vi "NATS READ.vi"(6 "timeout ms (conn default)":i32=-2, 7 "bytes to read (1024)":i32=1024, 8 "error in":errorcluster, 9 "reread on PING? (T)":bool=TRUE, 10 "suppress timeout error? (T)":bool=TRUE, 11 "nats connection in":T3={"connection ID"=refnum, "server INFO"="", "timeout ms"=5000, "verbose?"=FALSE, "server headers?"=FALSE, "client headers?"=FALSE}) -> (0 "error out":errorcluster, 1 "timeout?":bool, 2 "nats message":T1, 3 "nats connection out":T3={"connection ID"=refnum, "server INFO"="", "timeout ms"=5000, "verbose?"=FALSE, "server headers?"=FALSE, "client headers?"=FALSE})   [LabVIEW 2013, in "NATS Core.lvlib"]
doc: "Reads a message from the NATS server."
uses:
  NATS Core.lvlib
  Controls/nats connection.ctl
  Controls/nats message.ctl
  Controls/msg type.ctl
  <vilib>/dlg_ctls.llb/Space Constant.vi
  <vilib>/Utility/error.llb/Trim Whitespace.vi
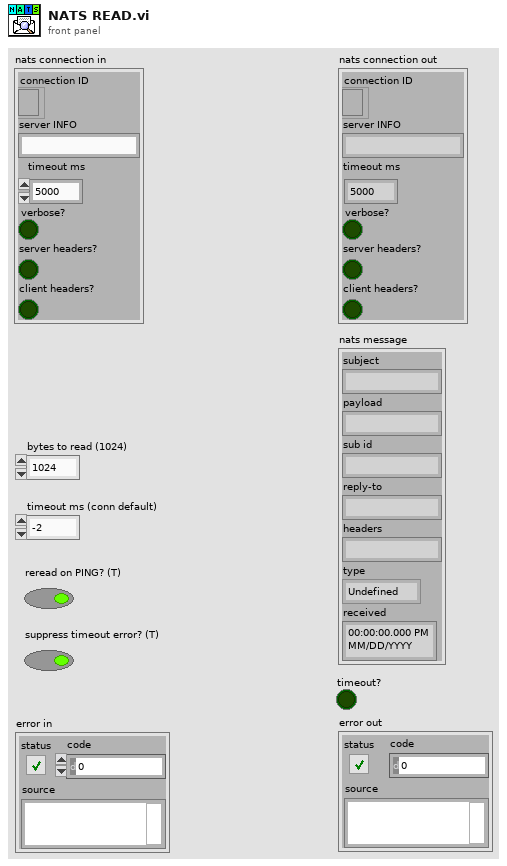
[diagram p1: front panel]
types:
  T1 = typedef "NATS Core.lvlib/nats message.ctl" = cluster{"subject":string, "payload":string, "sub id":string, "reply-to":string, "headers":string, "type":T2, "received":timestamp}
  T2 = typedef "NATS Core.lvlib/msg type.ctl" = enum16{"Undefined", "MSG", "HMSG", "+OK", "PING", "PONG", "-ERR", "INFO"}
  T3 = typedef "NATS Core.lvlib/nats connection.ctl" = cluster{"connection ID":refnum<k5>, "server INFO":string, "timeout ms":i32, "verbose?":bool, "server headers?":bool, "client headers?":bool}
  T4 = enum16{"Standard", "Buffered", "CRLF", "Immediate"}
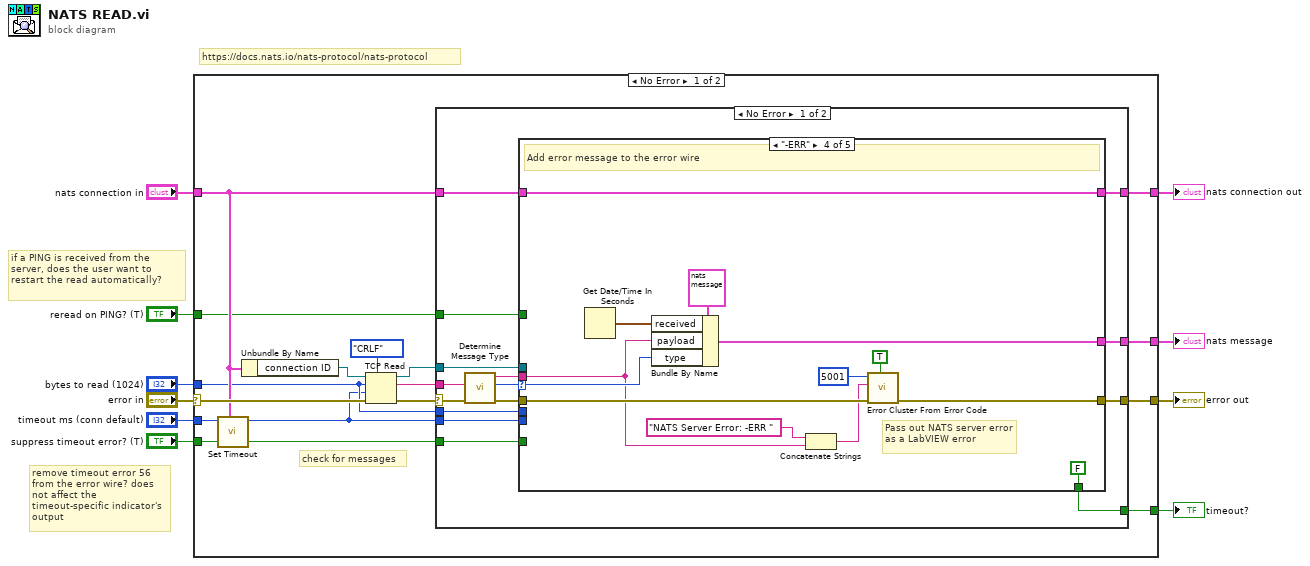
[diagram p0: block diagram]
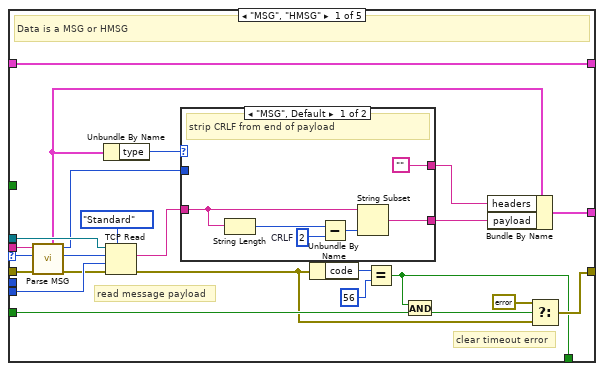
[diagram p2: hidden frame]
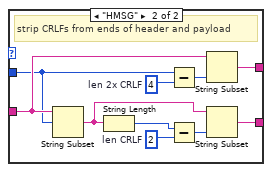
[diagram p3: hidden frame]
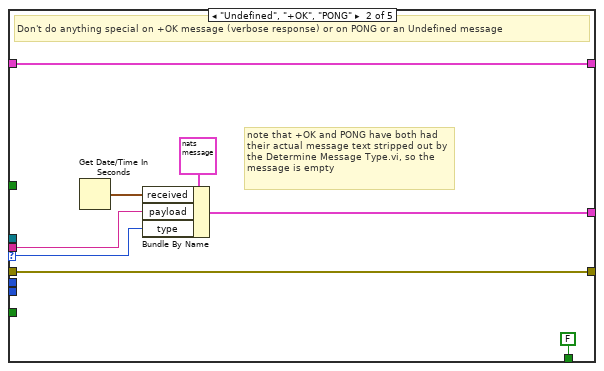
[diagram p4: hidden frame]
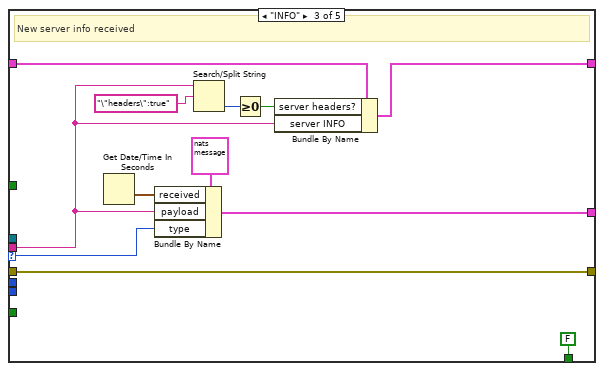
[diagram p5: hidden frame]
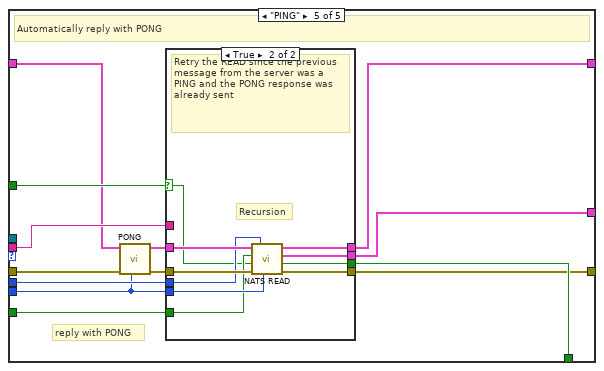
[diagram p6: hidden frame]
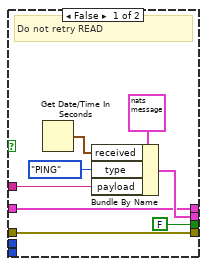
[diagram p7: hidden frame]
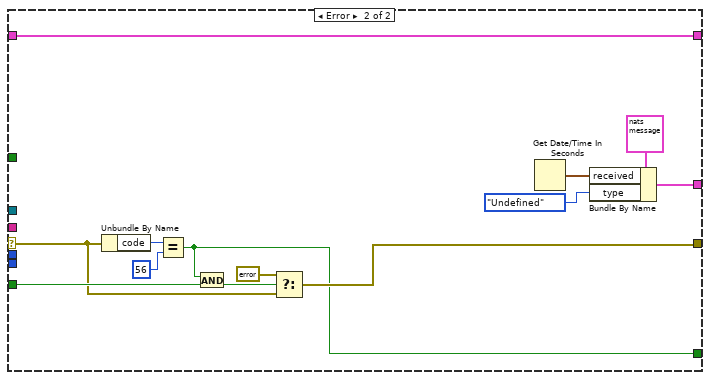
[diagram p8: hidden frame]
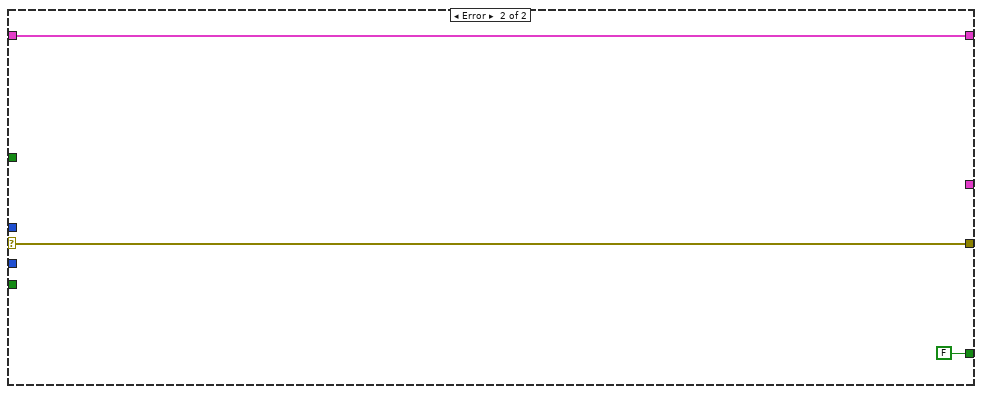
[diagram p9: hidden frame]
diagram:
  # "https://docs.nats.io/nats-protocol/nats-protocol"
  # "remove timeout error 56 from the error wire? does not affect the timeout-specific indicator's output"
  # "if a PING is received from the server, does the user want to restart the read automatically?"
  n1 = case shown="No Error" "error in" {
    selector: "error in" -> [w26 w161]
    tunnel: "nats connection in" -> [w17 w159]
    tunnel: [w24 w161] -> w8
    tunnel: "bytes to read (1024)" -> [w14 _]
    tunnel: "timeout ms (conn default)" -> [w18 _]
    tunnel: [w22 _] -> w5
    tunnel: [w21 FALSE ("specific error cleared?")] -> w4
    tunnel: [w19 w159] -> w3
    tunnel: "reread on PING? (T)" -> [w16 _]
    tunnel: "suppress timeout error? (T)" -> [w15 _]
    frame No Error {
      # "check for messages"
      n2 = call "Set Timeout.vi"("nats connection in"=w17, "timeout ms in"=w18) -> ("timeout ms out"=w13:i32)  [unwired: 9 in]
      n3 = Unbundle By Name(w17) -> ("connection ID"=w12:refnum<k5>)
      n4 = TCP Read(connection ID=w12, bytes to read=w14, error in (no error)=w26, 7:T4."CRLF" ("mode (standard)"), 9:w13) -> (connection ID out=w11:refnum<k5>, data out=w25:string, error out=w20:errorcluster)
      n5 = case shown="No Error" w20 {
        selector: w20 -> [w32 w148]
        tunnel: w25 -> [w33 _]
        tunnel: [w41 w147] -> w24
        tunnel: w13 -> [w40 _]
        tunnel: [w39 w154] -> w22
        tunnel: [w38 w146] -> w21
        tunnel: w17 -> [w37 w158]
        tunnel: [w36 w158] -> w19
        tunnel: w16 -> [w35 _]
        tunnel: w15 -> [w34 w149]
        tunnel: w14 -> [w28 _]
        tunnel: w11 -> [w27 _]
        frame No Error {
          n6 = call "Determine Message Type.vi"("error in"=w32, "data in"=w33) -> ("error out"=w31:errorcluster, "message type"=w30:T2, "stripped message"=w29:string)  [unwired: 7 in]
          n7 = case shown="\"-ERR\"" w30 {
            selector: w30 -> [w56 w88 w100 w113 _]
            tunnel: w31 -> [w53 w86 w98 w108 w118]
            tunnel: [w62 w86 w98 w107 w122] -> w41
            tunnel: w40 -> [w64 _ _ _ w115]
            tunnel: [w59 w87 w99 w112 w124] -> w39
            tunnel: [w43 FALSE ("timeout?") FALSE ("timeout?") FALSE ("timeout?") w123] -> w38
            tunnel: w37 -> [w60 w83 w90 w110 w119]
            tunnel: [w60 w83 w96 w110 w127] -> w36
            tunnel: w35 -> [_ _ _ _ w125]
            tunnel: w34 -> [w63 _ _ _ w121]
            tunnel: w29 -> [w61 w85 w93 w104 w120]
            tunnel: w28 -> [_ _ _ _ w126]
            tunnel: w27 -> [w54 _ _ _ _]
            frame "MSG", "HMSG" {
              # "clear timeout error"
              # "read message payload"
              # "Data is a MSG or HMSG"
              n8 = call "Parse MSG.vi"("error in"=w53, "message type"=w56, "stripped message"=w61) -> ("error out"=w52:errorcluster, "bytes to read"=w51:i32, "header length"=w48:i32, "nats message"=w49:T1)  [unwired: 5 in]
              n9 = Unbundle By Name(w49) -> ("type"=w50:T2)
              n10 = TCP Read(connection ID=w54, bytes to read=w51, error in (no error)=w52, 7:T4."Standard" ("mode (standard)"), 9:w64) -> (data out=w58:string, error out=w47:errorcluster)  [unwired: 1 out]
              n11 = case shown="\"MSG\", Default" w50 {
                tunnel: w58 -> [w69 w78]
                tunnel: w48 -> [_ w77]
                tunnel: ["" w79] -> w55
                tunnel: [w68 w74] -> w57
                frame "MSG", Default {
                  w67 = 2  # CRLF
                  # "strip CRLF from end of payload"
                  n12 = String Length(string=w69) -> (length=w66:i32)
                  n13 = Subtract(x=w66, y=w67) -> (x-y=w70:i32)
                  n14 = String Subset(string=w69, length (rest)=w70) -> (substring=w68:string)  [unwired: 1 in]
                }
                frame "HMSG" {
                  w76 = 2  # len CRLF
                  w80 = 4  # len 2x CRLF
                  # "strip CRLFs from ends of header and payload"
                  n15 = String Subset(string=w78, offset (0)=w77) -> (substring=w72:string)  [unwired: 1 in]
                  n16 = String Length(string=w72) -> (length=w73:i32)
                  n17 = Subtract(x=w77, y=w80) -> (x-y=w81:i32)
                  n18 = Subtract(x=w73, y=w76) -> (x-y=w75:i32)
                  n19 = String Subset(string=w78, length (rest)=w81) -> (substring=w79:string)  [unwired: 1 in]
                  n20 = String Subset(string=w72, length (rest)=w75) -> (substring=w74:string)  [unwired: 1 in]
                }
              }
              n21 = Unbundle By Name(w47) -> ("code"=w46:i32)
              n22 = Equal?(x=w46, y=56 ("timeout")) -> (x = y?=w43:bool)
              n23 = And(x=w43, y=w63) -> (x .and. y?=w44:bool)
              n24 = Bundle By Name(cluster=w49, "headers"=w55, "payload"=w57) -> (w59:T1)
              n25 = Select(t=errorcluster {"status"=FALSE, "code"=0, "source"=""}, s=w44, f=w47) -> (s? t:f=w62:errorcluster)
            }
            frame "Undefined", "+OK", "PONG" {
              # "note that +OK and PONG have both had their actual message text stripped out by the Determine Message Type.vi, so the message is empty"
              # "Don't do anything special on +OK message (verbose response) or on PONG or an Undefined message"
              n26 = Get Date/Time In Seconds() -> (seconds since 1Jan1904=w82:timestamp)
              n27 = Bundle By Name(cluster=T1 {"subject"="", "payload"="", "sub id"="", "reply-to"="", "headers"="", "type"=enum."Undefined", "received"=timestamp(0 s since 1904-01-01)} ("nats message"), "received"=w82, "payload"=w85, "type"=w88) -> (w87:T1)
            }
            frame "INFO" {
              # "New server info received"
              n28 = Get Date/Time In Seconds() -> (seconds since 1Jan1904=w95:timestamp)
              n29 = Bundle By Name(cluster=T1 {"subject"="", "payload"="", "sub id"="", "reply-to"="", "headers"="", "type"=enum."Undefined", "received"=timestamp(0 s since 1904-01-01)} ("nats message"), "received"=w95, "payload"=w93, "type"=w100) -> (w99:T1)
              n30 = Search/Split String(string=w93, search string/char (-)="\"headers\":true") -> (offset of match=w92:i32)  [unwired: 1 in, 2 out]
              n31 = Greater Or Equal To 0?(x=w92) -> (x >= 0?=w91:bool)
              n32 = Bundle By Name(cluster=w90, "server headers?"=w91, "server INFO"=w93) -> (w96:T3)
            }
            frame "-ERR" {
              # "Pass out NATS server error as a LabVIEW error"
              # "Add error message to the error wire"
              n33 = Get Date/Time In Seconds() -> (seconds since 1Jan1904=w106:timestamp)
              n34 = Bundle By Name(cluster=T1 {"subject"="", "payload"="", "sub id"="", "reply-to"="", "headers"="", "type"=enum."Undefined", "received"=timestamp(0 s since 1904-01-01)} ("nats message"), "received"=w106, "payload"=w104, "type"=w113) -> (w112:T1)
              n35 = Concatenate Strings("NATS Server Error: -ERR ", w104) -> (w103:string)
              n36 = call <vilib>:"Error Cluster From Error Code.vi"("show call chain? (False)"=TRUE, "error in (no error)"=w108, "error message (\"\")"=w103, "error code (0)"=5001) -> ("error out"=w107:errorcluster)  [unwired: 5 in]
            }
            frame "PING" {
              # "reply with PONG"
              # "Automatically reply with PONG"
              n37 = call "PONG.vi"("timeout ms (conn default)"=w115, "error in"=w118, "nats connection in"=w119) -> ("error out"=w116:errorcluster, "dup nats connection"=w117:T3)  [unwired: 7 in]
              n38 = case shown="True" w125 {
                selector: w125 -> [_ w136]
                tunnel: [w133 w140] -> w124
                tunnel: w116 -> [w131 w143]
                tunnel: w117 -> [w132 w145]
                tunnel: [w132 w144] -> w127
                tunnel: [w131 w142] -> w122
                tunnel: w115 -> [_ w141]
                tunnel: [FALSE ("timeout?") w139] -> w123
                tunnel: w126 -> [_ w138]
                tunnel: w121 -> [_ w137]
                tunnel: w120 -> [w129 _]
                frame False {
                  # "Do not retry READ"
                  n39 = Get Date/Time In Seconds() -> (seconds since 1Jan1904=w134:timestamp)
                  n40 = Bundle By Name(cluster=T1 {"subject"="", "payload"="", "sub id"="", "reply-to"="", "headers"="", "type"=enum."Undefined", "received"=timestamp(0 s since 1904-01-01)} ("nats message"), "received"=w134, "type"=msg_type."PING", "payload"=w129) -> (w133:T1)
                }
                frame True {
                  # "Recursion"
                  # "Retry the READ since the previous message from the server was a PING and the PONG response was already sent"
                  n41 = call "NATS READ.vi"("timeout ms (conn default)"=w141, "bytes to read (1024)"=w138, "error in"=w143, "reread on PING? (T)"=w136, "suppress timeout error? (T)"=w137, "nats connection in"=w145) -> ("error out"=w142:errorcluster, "timeout?"=w139:bool, "nats message"=w140:T1, "nats connection out"=w144:T3)  [unwired: 2 in]
                }
              }
            }
          }
        }
        frame Error {
          n42 = Unbundle By Name(w148) -> ("code"=w153:i32)
          n43 = Equal?(x=w153, y=56 ("timeout")) -> (x = y?=w146:bool)
          n44 = And(x=w146, y=w149) -> (x .and. y?=w151:bool)
          n45 = Select(t=errorcluster {"status"=FALSE, "code"=0, "source"=""}, s=w151, f=w148) -> (s? t:f=w147:errorcluster)
          n46 = Get Date/Time In Seconds() -> (seconds since 1Jan1904=w157:timestamp)
          n47 = Bundle By Name(cluster=T1 {"subject"="", "payload"="", "sub id"="", "reply-to"="", "headers"="", "type"=enum."Undefined", "received"=timestamp(0 s since 1904-01-01)} ("nats message"), "received"=w157, "type"=msg_type."Undefined" ("message type")) -> (w154:T1)
        }
      }
    }
    frame Error {
    }
  }
  "nats connection out" <- w3
  "error out" <- w8
  "nats message" <- w5
  "timeout?" <- w4
